vi "CaseStructure-Ver2.vi"() -> ()   [LabVIEW 2018]
panel:
  in  "OK Button":bool
  in  "?":bool
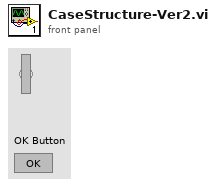
[diagram p1: front panel]
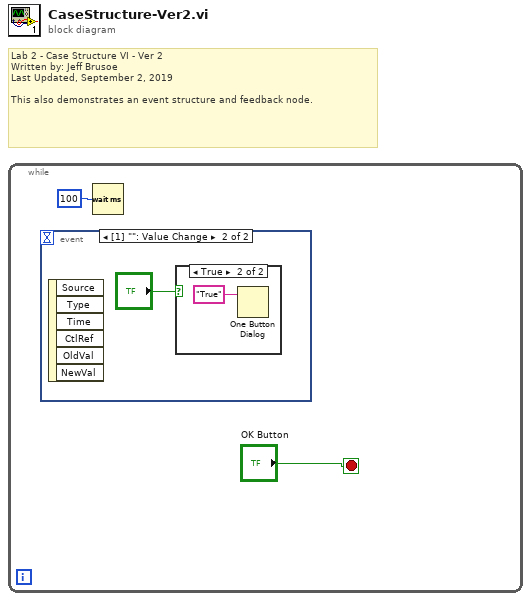
[diagram p0: block diagram]
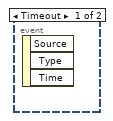
[diagram p2: hidden frame]
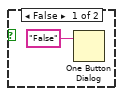
[diagram p3: hidden frame]
diagram:
  # "Lab 2 - Case Structure VI - Ver 2\nWritten by: Jeff Brusoe\nLast Updated, September 2, 2019\n\nThis also demonstrates an event structure and feedback node."
  n1 = while {
    stop <- "OK Button" stop-if-true
    n2 = event shown="[1] \"\": Value Change" {
      selector: _ -> [_ _]
      dyn-events: _ -> [_ _]
      timeout: _ -> [_ _]
      event Timeout {
        n3 = event-data() -> ()  [unwired: 1 in, 3 out]
      }
      event Value Change {
        n4 = event-data() -> ()  [unwired: 1 in, 6 out]
        n5 = case shown="True" "?" {
          frame False {
            n6 = One Button Dialog(message="False") -> ()  [unwired: 1 in, 1 out]
          }
          frame True {
            n7 = One Button Dialog(message="True") -> ()  [unwired: 1 in, 1 out]
          }
        }
      }
    }
    n8 = Wait (ms)(milliseconds to wait=100) -> ()  [unwired: 1 out]
  }
